vi "OpenTDMS.vi"(10 "Data In":T1={"DAQ Config Data"={"Vertical"={"Coupling"=1, "Offset (V)"=-0.5, "Range (V)"=2.0, "Impedance"=50.0}, "Horizontal"={"Offset Time"=0.0, "Sample Time (S)"=22.0, "Sample Points"=1000}, "Trigger\n"={"Lower Level (V)"=-0.02, "Trigger Slope"=1, "Trigger Source"=10}, "Acquisition"={"Trigger Mode"=1, "Initiate Continuously"=0, "Acquire Type"=0, "Acquire Count"=1}, "Channel"=0, "Instrument Handle"=0, "Error"={"status"=FALSE, "code"=0, "source"=""}, "State"=1}, "Acquisition"={"Current"={"Acquiring Now?"=FALSE, "Waveforms Acquired"=0.0, "Start of Acquisition"=timestamp(0 s since 1904-01-01), "Acquisition Name"=""}, "Stop Condition"={"Quota"=3000.0, "Duration (S)"=22, "Stop Condition"=FALSE}, "Config Needed"=FALSE}, "Measurement"={"Waveform"={"t0"=timestamp(0 s since 1904-01-01), "dt"=1.0, "Y"=[]}, "Peak Heights"=[], "Acquisition Time"=timestamp(0 s since 1904-01-01), "File Path"=path "C:/Users/lab-341/Desktop/Reed/Oscilloscope VI/pulses.tdms", "TDMS File Handle"=refnum}, "UI References"={"Acquire"=refnum, "Configure DAQ"=refnum, "Measurement (Ch1)"=refnum, "Update Needed?"=FALSE, "New Run"=refnum, "Signal"=refnum}, "Run Info"={"Active Run?"=FALSE, "Run Notes"="Enter in notes explaining the purpose of the run and any unusual steps taken in the process. This should make it clear why the data was taken. e.g. \"Measuring LXe scintillation light with Teflon\" or \"Measuring dark pulses to determine SPE gain.\" Concise is good but precise is better.", "User Name"="", "Campaign ID#"="", "Run Name"="", "Start Time"=timestamp(0 s since 1904-01-01), "End Time"=timestamp(0 s since 1904-01-01)}, "System Status"={"Bias Voltage"=0.0, "SiPM Temperature"=[], "Slow Control User"="", "LXe"=0.0}, "Acquisition Info"={"Trigger Mode"=FALSE, "Acquisition Mode"=FALSE, "Bias Voltage (V)"=0.0, "Preamplifier"=0, "Shaping Amplifier"=0, "Acquisition Notes"="", "1"=FALSE, "2"=FALSE}} {"Acquisition Info"."Shaping Amplifier" items=["CR-200-100ns", "CR-200-1us"]; "Acquisition Info"."Preamplifier" items=["CR-Z-113-1k", "CR-Z-113-5k", "CR-Z-SiPM"]; "DAQ Config Data"."State" items=["Enable"=1, "Disable"=0]; "DAQ Config Data"."Channel" items=["Input Channel 1", "Input Channel 2", "Input Channel 3", "Input Channel 4"]; "DAQ Config Data"."Acquisition"."Acquire Type" items=["Normal"=0, "Average"=1, "Envelope"=2, "Peak Detect"=3, "High Resolution"=4, "Fast"=5, "Equivalent Time"=16]; "DAQ Config Data"."Acquisition"."Initiate Continuously" items=["Continuously"=1, "Single Capture"=0]; "DAQ Config Data"."Acquisition"."Trigger Mode" items=["Auto", "Normal"]; "DAQ Config Data"."Trigger"."Trigger Source" items=["TTL0", "TTL1", "TTL2", "TTL3", "TTL4", "TTL5", "TTL6", "TTL7", "ECL0", "ECL1", "Input Channel 1", "Input Channel 2", "Input Channel 3", "Input Channel 4", "External Trigger Source", "STAR", "Manual Trigger", "Pattern"]; "DAQ Config Data"."Trigger"."Trigger Slope" items=["Rising Edge", "Falling Edge"]; "DAQ Config Data"."Horizontal"."Sample Time (S)" items=["0.5"=0.5, "0.4"=0.4, "0.25"=0.25, "0.2"=0.2, "0.1"=0.1, "0.05"=0.05, "0.04"=0.04, "0.025"=0.025, "0.02"=0.02, "0.01"=0.01, "0.005"=0.005, "0.004"=0.004, "0.0025"=0.0025, "0.002"=0.002, "0.001"=0.001, "5E-4"=0.0005, "4E-4"=0.0004, "2.5E-4"=0.00025, "2E-4"=0.0002, "1E-4"=0.0001, "5E-5"=5e-05, "4E-5"=4e-05, "2E-5"=2e-05, "5E-6"=5e-06, "1E-6"=1e-06, "5E-7"=5e-07, "1E-7"=1e-07, "5E-8"=5e-08, "1E-8"=1e-08]; "DAQ Config Data"."Vertical"."Impedance" items=["50 Ohm"=50.0, "1 MOhm"=1000000.0]; "DAQ Config Data"."Vertical"."Range (V)" items=["10"=10.0, "5"=5.0, "2"=2.0, "1"=1.0, "0.4"=0.4, "0.2"=0.2, "0.08"=0.08, "0.04"=0.04, "0.02"=0.02, "0.01"=0.01]; "DAQ Config Data"."Vertical"."Coupling" items=["AC", "DC"]}) -> (3 "Data Out":T1={"DAQ Config Data"={"Vertical"={"Coupling"=1, "Offset (V)"=-0.5, "Range (V)"=2.0, "Impedance"=50.0}, "Horizontal"={"Offset Time"=0.0, "Sample Time (S)"=22.0, "Sample Points"=1000}, "Trigger\n"={"Lower Level (V)"=-0.02, "Trigger Slope"=1, "Trigger Source"=10}, "Acquisition"={"Trigger Mode"=1, "Initiate Continuously"=0, "Acquire Type"=0, "Acquire Count"=1}, "Channel"=0, "Instrument Handle"=0, "Error"={"status"=FALSE, "code"=0, "source"=""}, "State"=1}, "Acquisition"={"Current"={"Acquiring Now?"=FALSE, "Waveforms Acquired"=0.0, "Start of Acquisition"=timestamp(0 s since 1904-01-01), "Acquisition Name"=""}, "Stop Condition"={"Quota"=3000.0, "Duration (S)"=22, "Stop Condition"=FALSE}, "Config Needed"=FALSE}, "Measurement"={"Waveform"={"t0"=timestamp(0 s since 1904-01-01), "dt"=1.0, "Y"=[]}, "Peak Heights"=[], "Acquisition Time"=timestamp(0 s since 1904-01-01), "File Path"=path "C:/Users/lab-341/Desktop/Reed/Oscilloscope VI/pulses.tdms", "TDMS File Handle"=refnum}, "UI References"={"Acquire"=refnum, "Configure DAQ"=refnum, "Measurement (Ch1)"=refnum, "Update Needed?"=FALSE, "New Run"=refnum, "Signal"=refnum}, "Run Info"={"Active Run?"=FALSE, "Run Notes"="Enter in notes explaining the purpose of the run and any unusual steps taken in the process. This should make it clear why the data was taken. e.g. \"Measuring LXe scintillation light with Teflon\" or \"Measuring dark pulses to determine SPE gain.\" Concise is good but precise is better.", "User Name"="", "Campaign ID#"="", "Run Name"="", "Start Time"=timestamp(0 s since 1904-01-01), "End Time"=timestamp(0 s since 1904-01-01)}, "System Status"={"Bias Voltage"=0.0, "SiPM Temperature"=[], "Slow Control User"="", "LXe"=0.0}, "Acquisition Info"={"Trigger Mode"=FALSE, "Acquisition Mode"=FALSE, "Bias Voltage (V)"=0.0, "Preamplifier"=0, "Shaping Amplifier"=0, "Acquisition Notes"="", "1"=FALSE, "2"=FALSE}} {"Acquisition Info"."Shaping Amplifier" items=["CR-200-100ns", "CR-200-1us"]; "Acquisition Info"."Preamplifier" items=["CR-Z-113-1k", "CR-Z-113-5k", "CR-Z-SiPM"]; "DAQ Config Data"."State" items=["Enable"=1, "Disable"=0]; "DAQ Config Data"."Channel" items=["Input Channel 1", "Input Channel 2", "Input Channel 3", "Input Channel 4"]; "DAQ Config Data"."Acquisition"."Acquire Type" items=["Normal"=0, "Average"=1, "Envelope"=2, "Peak Detect"=3, "High Resolution"=4, "Fast"=5, "Equivalent Time"=16]; "DAQ Config Data"."Acquisition"."Initiate Continuously" items=["Continuously"=1, "Single Capture"=0]; "DAQ Config Data"."Acquisition"."Trigger Mode" items=["Auto", "Normal"]; "DAQ Config Data"."Trigger"."Trigger Source" items=["TTL0", "TTL1", "TTL2", "TTL3", "TTL4", "TTL5", "TTL6", "TTL7", "ECL0", "ECL1", "Input Channel 1", "Input Channel 2", "Input Channel 3", "Input Channel 4", "External Trigger Source", "STAR", "Manual Trigger", "Pattern"]; "DAQ Config Data"."Trigger"."Trigger Slope" items=["Rising Edge", "Falling Edge"]; "DAQ Config Data"."Horizontal"."Sample Time (S)" items=["0.5"=0.5, "0.4"=0.4, "0.25"=0.25, "0.2"=0.2, "0.1"=0.1, "0.05"=0.05, "0.04"=0.04, "0.025"=0.025, "0.02"=0.02, "0.01"=0.01, "0.005"=0.005, "0.004"=0.004, "0.0025"=0.0025, "0.002"=0.002, "0.001"=0.001, "5E-4"=0.0005, "4E-4"=0.0004, "2.5E-4"=0.00025, "2E-4"=0.0002, "1E-4"=0.0001, "5E-5"=5e-05, "4E-5"=4e-05, "2E-5"=2e-05, "5E-6"=5e-06, "1E-6"=1e-06, "5E-7"=5e-07, "1E-7"=1e-07, "5E-8"=5e-08, "1E-8"=1e-08]; "DAQ Config Data"."Vertical"."Impedance" items=["50 Ohm"=50.0, "1 MOhm"=1000000.0]; "DAQ Config Data"."Vertical"."Range (V)" items=["10"=10.0, "5"=5.0, "2"=2.0, "1"=1.0, "0.4"=0.4, "0.2"=0.2, "0.08"=0.08, "0.04"=0.04, "0.02"=0.02, "0.01"=0.01]; "DAQ Config Data"."Vertical"."Coupling" items=["AC", "DC"]})   [LabVIEW 2012]
uses:
  Oscilloscope/TypeDefs/DataTypes/Data.ctl
  Oscilloscope/TypeDefs/DataTypes/DAQConfig.ctl
  Oscilloscope/TypeDefs/DataTypes/Acquisition.ctl
  Oscilloscope/TypeDefs/DataTypes/Current.ctl
  Oscilloscope/TypeDefs/DataTypes/StopCondition.ctl
  Oscilloscope/TypeDefs/DataTypes/Measurement.ctl
  Oscilloscope/TypeDefs/DataTypes/UIReferences.ctl
  Oscilloscope/TypeDefs/DataTypes/RunInfo.ctl
  TypeDefs/DataTypes/SystemStatus.ctl
panel:
  # "Shaper Gain"
  # "Self"
  # "Fast"
  # "Solicited"
  # "Standard"
  # "Shaper Gain"
  # "Self"
  # "Fast"
  # "Solicited"
  # "Standard"
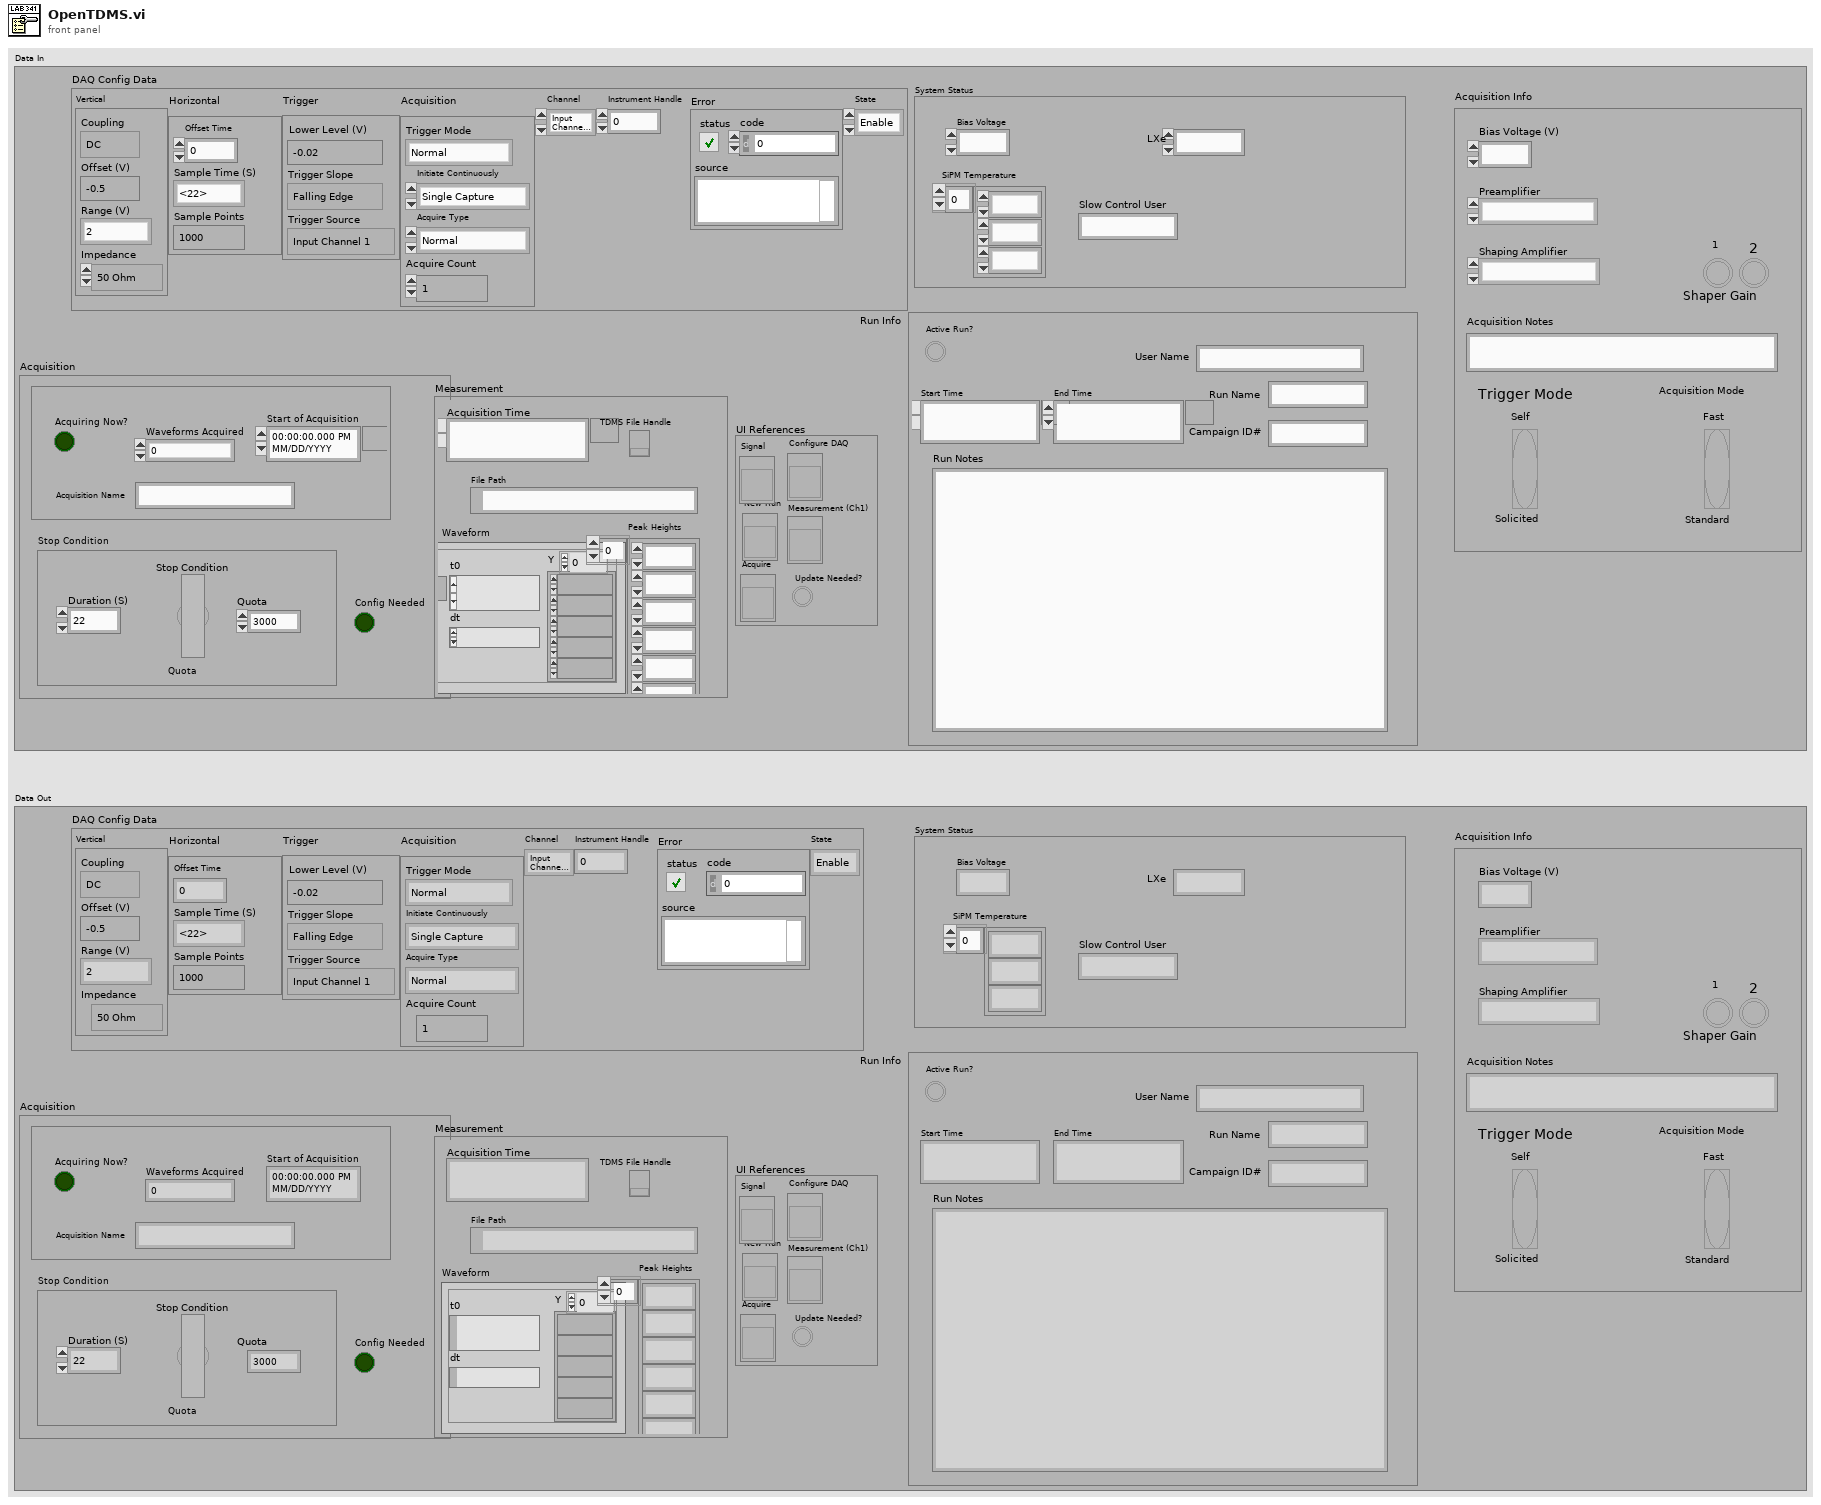
[diagram p1: front panel]
types:
  T1 = typedef "Data.ctl" = cluster{"DAQ Config Data":T2, "Acquisition":T3, "Measurement":T6, "UI References":T7, "Run Info":T8, "System Status":T9, "Acquisition Info":cluster{"Trigger Mode":bool, "Acquisition Mode":bool, "Bias Voltage (V)":dbl, "Preamplifier":u16, "Shaping Amplifier":u16, "Acquisition Notes":string, "1":bool, "2":bool}}
  T2 = typedef "DAQConfig.ctl" = cluster{"Vertical":cluster{"Coupling":i32, "Offset (V)":dbl, "Range (V)":dbl, "Impedance":dbl}, "Horizontal":cluster{"Offset Time":dbl, "Sample Time (S)":dbl, "Sample Points":u32}, "Trigger\n":cluster{"Lower Level (V)":dbl, "Trigger Slope":i32, "Trigger Source":i32}, "Acquisition":cluster{"Trigger Mode":i32, "Initiate Continuously":i32, "Acquire Type":i32, "Acquire Count":i32}, "Channel":i32, "Instrument Handle":i32, "Error":errorcluster, "State":i32}
  T3 = typedef "Acquisition.ctl" = cluster{"Current":T4, "Stop Condition":T5, "Config Needed":bool}
  T4 = typedef "Current.ctl" = cluster{"Acquiring Now?":bool, "Waveforms Acquired":dbl, "Start of Acquisition":timestamp, "Acquisition Name":string}
  T5 = typedef "StopCondition.ctl" = cluster{"Quota":dbl, "Duration (S)":u16, "Stop Condition":bool}
  T6 = typedef "Measurement.ctl" = cluster{"Waveform":waveform(dbl), "Peak Heights":dbl[], "Acquisition Time":timestamp, "File Path":path, "TDMS File Handle":refnum<k34>}
  T7 = typedef "UIReferences.ctl" = cluster{"Acquire":refnum<vi>, "Configure DAQ":refnum<vi>, "Measurement (Ch1)":refnum<vi>, "Update Needed?":bool, "New Run":refnum<vi>, "Signal":refnum<vi>}
  T8 = typedef "RunInfo.ctl" = cluster{"Active Run?":bool, "Run Notes":string, "User Name":string, "Campaign ID#":string, "Run Name":string, "Start Time":timestamp, "End Time":timestamp}
  T9 = typedef "SystemStatus.ctl" = cluster{"Bias Voltage":dbl, "SiPM Temperature":dbl[], "Slow Control User":string, "LXe":dbl}
  T10 = enum16{"open", "open or create", "create or replace", "create", "open (read-only)"}
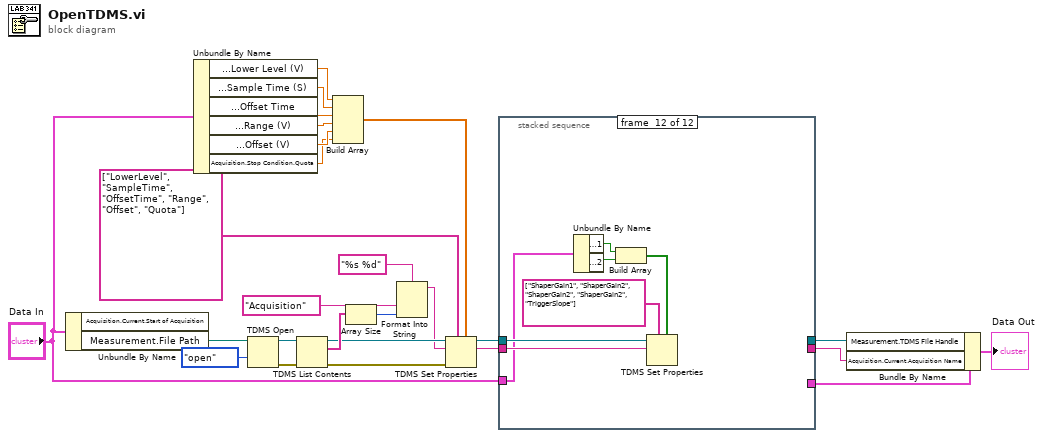
[diagram p0: block diagram]
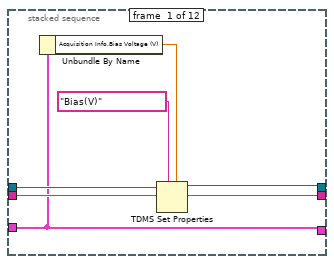
[diagram p2: hidden frame]
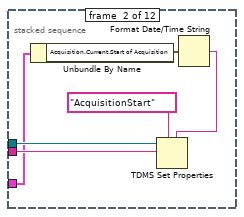
[diagram p3: hidden frame]
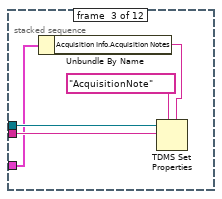
[diagram p4: hidden frame]
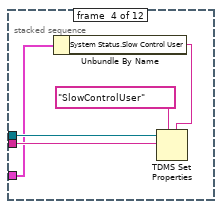
[diagram p5: hidden frame]
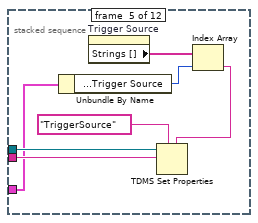
[diagram p6: hidden frame]
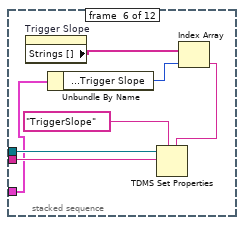
[diagram p7: hidden frame]
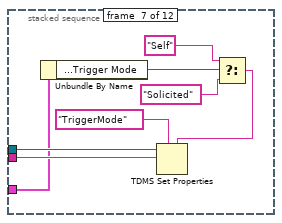
[diagram p8: hidden frame]
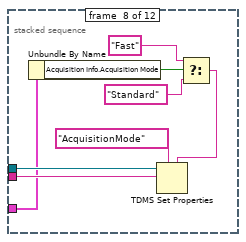
[diagram p9: hidden frame]
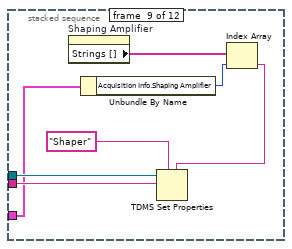
[diagram p10: hidden frame]
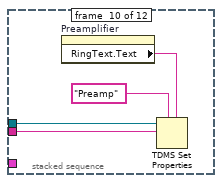
[diagram p11: hidden frame]
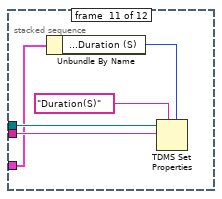
[diagram p12: hidden frame]
diagram:
  n1 = Unbundle By Name("Data In") -> ("Measurement.File Path"=w17:path)  [unwired: 1 out]
  n2 = Unbundle By Name("Data In") -> ("DAQ Config Data.Trigger.Lower Level (V)"=w24:dbl, "DAQ Config Data.Horizontal.Sample Time (S)"=w23:dbl, "DAQ Config Data.Horizontal.Offset Time"=w22:dbl, "DAQ Config Data.Vertical.Range (V)"=w21:dbl, "DAQ Config Data.Vertical.Offset (V)"=w20:dbl, "Acquisition.Stop Condition.Quota"=w7:dbl)
  n3 = TDMS Open(10:T10."open" ("operation (0:open)"), 11:w17) -> (0:w14:errorcluster, 3:w15:refnum<k34>)  [unwired: 4 in]
  n4 = TDMS List Contents(4:w14, 7:w15) -> (0:w9:errorcluster, 2:w16:string[], 3:w10:refnum<k34>)  [unwired: 1 in, 1 out]
  n5 = Build Array(w24, w23, w22, w21, w20, w7) -> (w19:dbl[])
  n6 = Array Size(array=w16) -> (size(s)=w13:i32)
  n7 = Format Into String(format string="%s %d", "Acquisition" ("group name in (Untitled)"), w13) -> (resulting string=w8:string)  [unwired: 2 in, 1 out]
  n8 = TDMS Set Properties(5:w19, 7:string[] ["LowerLevel", "SampleTime", "OffsetTime", "Range", "Offset", "Quota"] ("property names"), 8:w9, 10:w8, 11:w10) -> (2:w4:string, 3:w5:refnum<k34>)  [unwired: 1 in, 2 out]
  n9 = stacked-sequence {
    tunnel: "Data In" -> [w27 w34 w40 w46 w50 w58 w68 w76 w80 _ w91 w100]
    tunnel: [w27 _ _ _ _ _ _ _ _ _ _ _] -> w6
    tunnel: w5 -> [w33 w39 w44 w49 w56 w63 w71 w79 w82 w90 w95 w102]
    tunnel: [w31 _ _ _ _ _ _ _ _ _ _ _] -> w2
    tunnel: [w30 _ _ _ _ _ _ _ _ _ _ _] -> w1
    tunnel: w4 -> [w32 w38 w43 w48 w55 w62 w70 w78 w86 w89 w94 w101]
    frame #0 {
      n10 = Unbundle By Name(w27) -> ("Acquisition Info.Bias Voltage (V)"=w29:dbl)
      n11 = TDMS Set Properties(5:w29, 7:"Bias(V)", 10:w32, 11:w33) -> (2:w30:string, 3:w31:refnum<k34>)  [unwired: 2 in, 2 out]
    }
    frame #1 {
      n12 = Unbundle By Name(w34) -> ("Acquisition.Current.Start of Acquisition"=w36:timestamp)
      n13 = Format Date/Time String(seconds (now)=w36) -> (date/time string=w35:string)  [unwired: 2 in]
      n14 = TDMS Set Properties(5:w35, 7:"AcquisitionStart", 10:w38, 11:w39) -> ()  [unwired: 2 in, 4 out]
    }
    frame #2 {
      n15 = Unbundle By Name(w40) -> ("Acquisition Info.Acquisition Notes"=w41:string)
      n16 = TDMS Set Properties(5:w41, 7:"AcquisitionNote", 10:w43, 11:w44) -> ()  [unwired: 2 in, 4 out]
    }
    frame #3 {
      n17 = Unbundle By Name(w46) -> ("System Status.Slow Control User"=w45:string)
      n18 = TDMS Set Properties(5:w45, 7:"SlowControlUser", 10:w48, 11:w49) -> ()  [unwired: 2 in, 4 out]
    }
    frame #4 {
      n19 = Unbundle By Name(w50) -> ("DAQ Config Data.Trigger.Trigger Source"=w54:i32)
      n20 = property on="Trigger Source" class="Ring (strict)"() -> ("Strings []"=w53:string[])  [unwired: 2 in, 2 out]
      n21 = Index Array(array=w53, index=w54) -> (element=w52:string)
      n22 = TDMS Set Properties(5:w52, 7:"TriggerSource", 10:w55, 11:w56) -> ()  [unwired: 2 in, 4 out]
    }
    frame #5 {
      n23 = property on="Trigger Slope" class="Ring (strict)"() -> ("Strings []"=w57:string[])  [unwired: 2 in, 2 out]
      n24 = Unbundle By Name(w58) -> ("DAQ Config Data.Trigger.Trigger Slope"=w61:i32)
      n25 = Index Array(array=w57, index=w61) -> (element=w60:string)
      n26 = TDMS Set Properties(5:w60, 7:"TriggerSlope", 10:w62, 11:w63) -> ()  [unwired: 2 in, 4 out]
    }
    frame #6 {
      n27 = Unbundle By Name(w68) -> ("Acquisition Info.Trigger Mode"=w65:bool)
      n28 = Select(t="Self", s=w65, f="Solicited") -> (s? t:f=w64:string)
      n29 = TDMS Set Properties(5:w64, 7:"TriggerMode", 10:w70, 11:w71) -> ()  [unwired: 2 in, 4 out]
    }
    frame #7 {
      n30 = Unbundle By Name(w76) -> ("Acquisition Info.Acquisition Mode"=w75:bool)
      n31 = Select(t="Fast", s=w75, f="Standard") -> (s? t:f=w72:string)
      n32 = TDMS Set Properties(5:w72, 7:"AcquisitionMode", 10:w78, 11:w79) -> ()  [unwired: 2 in, 4 out]
    }
    frame #8 {
      n33 = property on="Shaping Amplifier" class="Ring (strict)"() -> ("Strings []"=w85:string[])  [unwired: 2 in, 2 out]
      n34 = Unbundle By Name(w80) -> ("Acquisition Info.Shaping Amplifier"=w84:u16)
      n35 = Index Array(array=w85, index=w84) -> (element=w83:string)
      n36 = TDMS Set Properties(5:w83, 7:"Shaper", 10:w86, 11:w82) -> ()  [unwired: 2 in, 4 out]
    }
    frame #9 {
      n37 = property on="Preamplifier" class="Ring (strict)"() -> ("RingText.Text"=w87:string)  [unwired: 2 in, 2 out]
      n38 = TDMS Set Properties(5:w87, 7:"Preamp", 10:w89, 11:w90) -> ()  [unwired: 2 in, 4 out]
    }
    frame #10 {
      n39 = Unbundle By Name(w91) -> ("Acquisition.Stop Condition.Duration (S)"=w92:u16)
      n40 = TDMS Set Properties(5:w92, 7:"Duration(S)", 10:w94, 11:w95) -> ()  [unwired: 2 in, 4 out]
    }
    frame #11 {
      n41 = Unbundle By Name(w100) -> ("Acquisition Info.1"=w99:bool, "Acquisition Info.2"=w98:bool)
      n42 = Build Array(w99, w98) -> (w97:bool[])
      n43 = TDMS Set Properties(5:w97, 7:string[] ["ShaperGain1", "ShaperGain2", "ShaperGain2", "ShaperGain2", "TriggerSlope"] ("property names"), 10:w101, 11:w102) -> ()  [unwired: 2 in, 4 out]
    }
  }
  n44 = Bundle By Name(cluster=w6, "Measurement.TDMS File Handle"=w2, "Acquisition.Current.Acquisition Name"=w1) -> (→"Data Out":T1)
